vi "ICS425 Data Parse.vi"(8 "Error In":errorcluster, 10 "Input Data":string=" -17.804  PS\r\n") -> (0 "Error Out":errorcluster, 2 "Output Data":string=" -17.804  PS\r\n", 4 "Data & Stability":bool, 6 "Weight":dbl)   [LabVIEW 2018]
uses:
  <vilib>/Utility/error.llb/whitespace.ctl
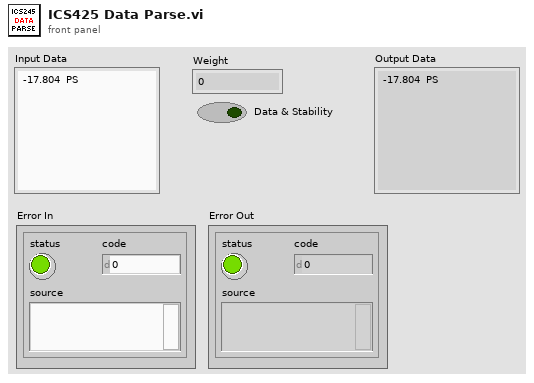
[diagram p1: front panel]
types:
  T1 = typedef "whitespace.ctl" = u16
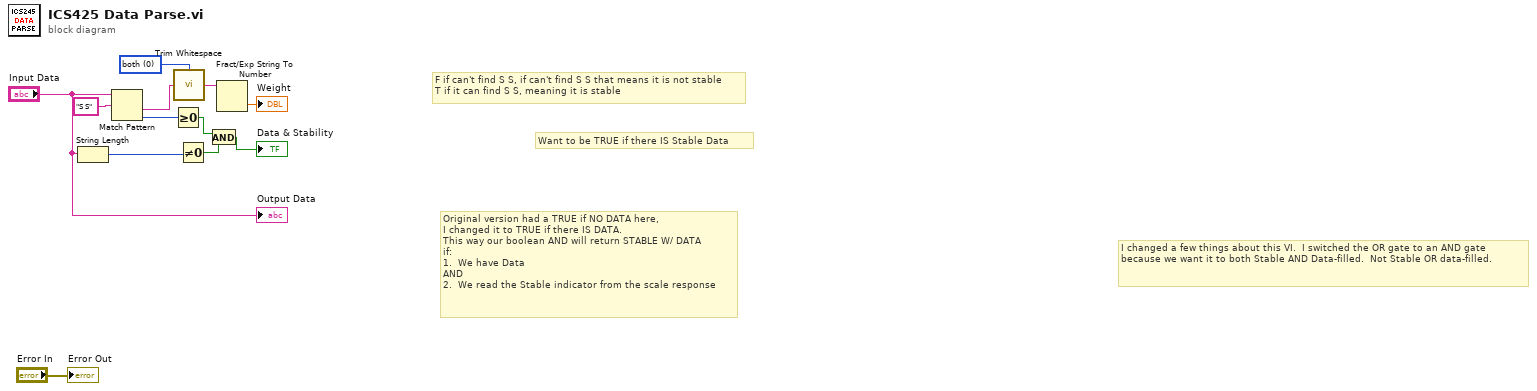
[diagram p0: block diagram]
diagram:
  w8 = T1 0 items=["both", "start of string", "end of string"] ("location (both)")
  # "I changed a few things about this VI.  I switched the OR gate to an AND gate\nbecause we want it to both Stable AND Data-filled.  Not Stable OR data-filled."
  # "Want to be TRUE if there IS Stable Data"
  # "F if can't find S S, if can't find S S that means it is not stable\nT if it can find S S, meaning it is stable"
  # "Original version had a TRUE if NO DATA here,\nI changed it to TRUE if there IS DATA.  \nThis way our boolean AND will return STABLE W/ DATA\nif:\n1.  We have Data\nAND\n2.  We read the Stable indicator from the scale response"
  n1 = String Length(string="Input Data") -> (length=w1:i32)
  n2 = Match Pattern(string="Input Data", regular expression="S S") -> (after substring=w5:string, offset past match=w12:i32)  [unwired: 1 in, 2 out]
  n3 = Greater Or Equal To 0?(x=w12) -> (x >= 0?=w4:bool)
  n4 = call <vilib>:"Trim Whitespace.vi"("string"=w5, "location (both)"=w8) -> ("trimmed string"=w7:string)
  n5 = Not Equal To 0?(x=w1) -> (x != 0?=w2:bool)
  n6 = And(x=w4, y=w2) -> (x .and. y?=→"Data & Stability":bool)
  n7 = Fract/Exp String To Number(string=w7) -> (number=→"Weight":dbl)  [unwired: 3 in, 1 out]
  "Error Out" <- "Error In"
  "Output Data" <- "Input Data"
